vi "RichToFlatrfcontrol_ControlParams.vi"(5 "OutputClusterType":T1, 11 "InputCluster":T2) -> (3 "OutputCluster":T1)   [LabVIEW 2024, in "FlexCompute_grpc_client.lvlib"]
uses:
  FlexCompute_grpc_client.lvlib
  rfcontrol_ControlParams.ctl
  rfcontrol_ControlParams_Flat.ctl
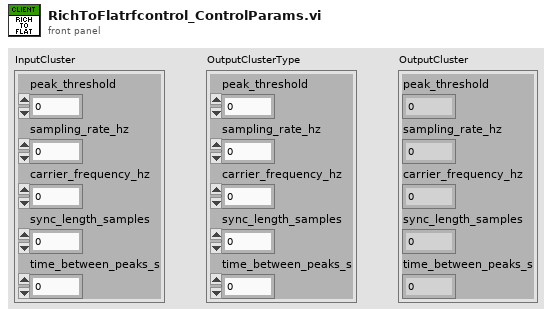
[diagram p1: front panel]
types:
  T1 = typedef "FlexCompute_grpc_client.lvlib/rfcontrol_ControlParams_Flat.ctl" = cluster{"peak_threshold":dbl, "sampling_rate_hz":dbl, "carrier_frequency_hz":dbl, "sync_length_samples":u32, "time_between_peaks_s":dbl}
  T2 = typedef "FlexCompute_grpc_client.lvlib/rfcontrol_ControlParams.ctl" = cluster{"peak_threshold":dbl, "sampling_rate_hz":dbl, "carrier_frequency_hz":dbl, "sync_length_samples":u32, "time_between_peaks_s":dbl}
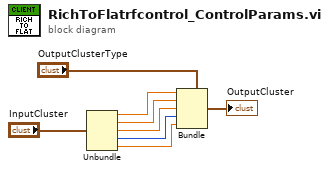
[diagram p0: block diagram]
diagram:
  n1 = Unbundle "Unbundle"("InputCluster") -> ("peak_threshold"=w5:dbl, "sampling_rate_hz"=w4:dbl, "carrier_frequency_hz"=w3:dbl, "sync_length_samples"=w2:u32, "time_between_peaks_s"=w1:dbl)
  n2 = Bundle "Bundle"(cluster="OutputClusterType", "peak_threshold"=w5, "sampling_rate_hz"=w4, "carrier_frequency_hz"=w3, "sync_length_samples"=w2, "time_between_peaks_s"=w1) -> (→"OutputCluster":T1)
